vi "Read Single Point.vi"(8 "error in (no error)":errorcluster, 11 "Simulated DMM in":refnum<class "Simulated DMM.lvclass">) -> (0 "error out":errorcluster, 2 "Measurement":dbl, 3 "Simulated DMM out":refnum<class "Simulated DMM.lvclass">)   [LabVIEW 2017, in "Simulated DMM.lvclass"]
uses:
  Simulated DMM.lvclass
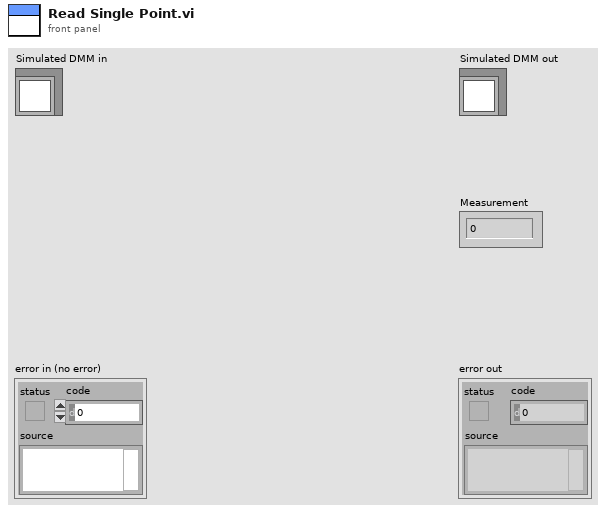
[diagram p1: front panel]
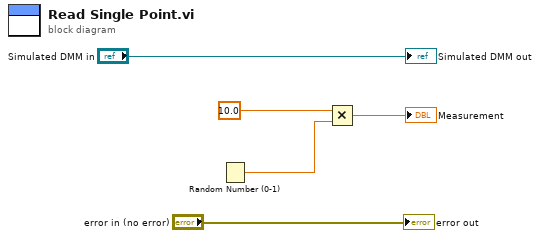
[diagram p0: block diagram]
diagram:
  n1 = Random Number (0-1)() -> (number: 0 to 1=w3:dbl)
  n2 = Multiply(x=10.0, y=w3) -> (x*y=→"Measurement":dbl)
  "error out" <- "error in (no error)"
  "Simulated DMM out" <- "Simulated DMM in"
